vi "加标模块单控对话框.vi"(10 "数组":refnum<vi>[](array[refnum]), 11 "标题":string="加标模块") -> ()   [LabVIEW 2016, in "质控单元.lvlib"]
panel:
  in  "慢速到液位":bool
  in  "排液":bool
  in  "退出":bool
  in  "柱塞泵":bool
  in  "排液":bool
  in  "搅拌":bool
  in  "进样调速":bool
  in  "进样":bool
  in  "停止":bool
  in  "加标启动":bool
  # "手动控制"
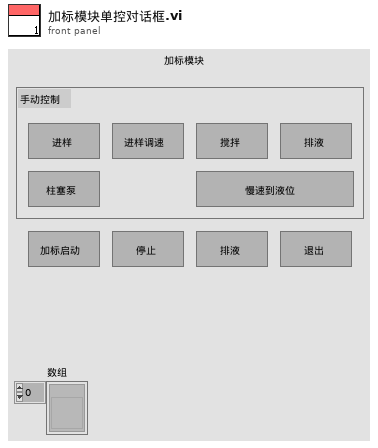
[diagram p1: front panel]
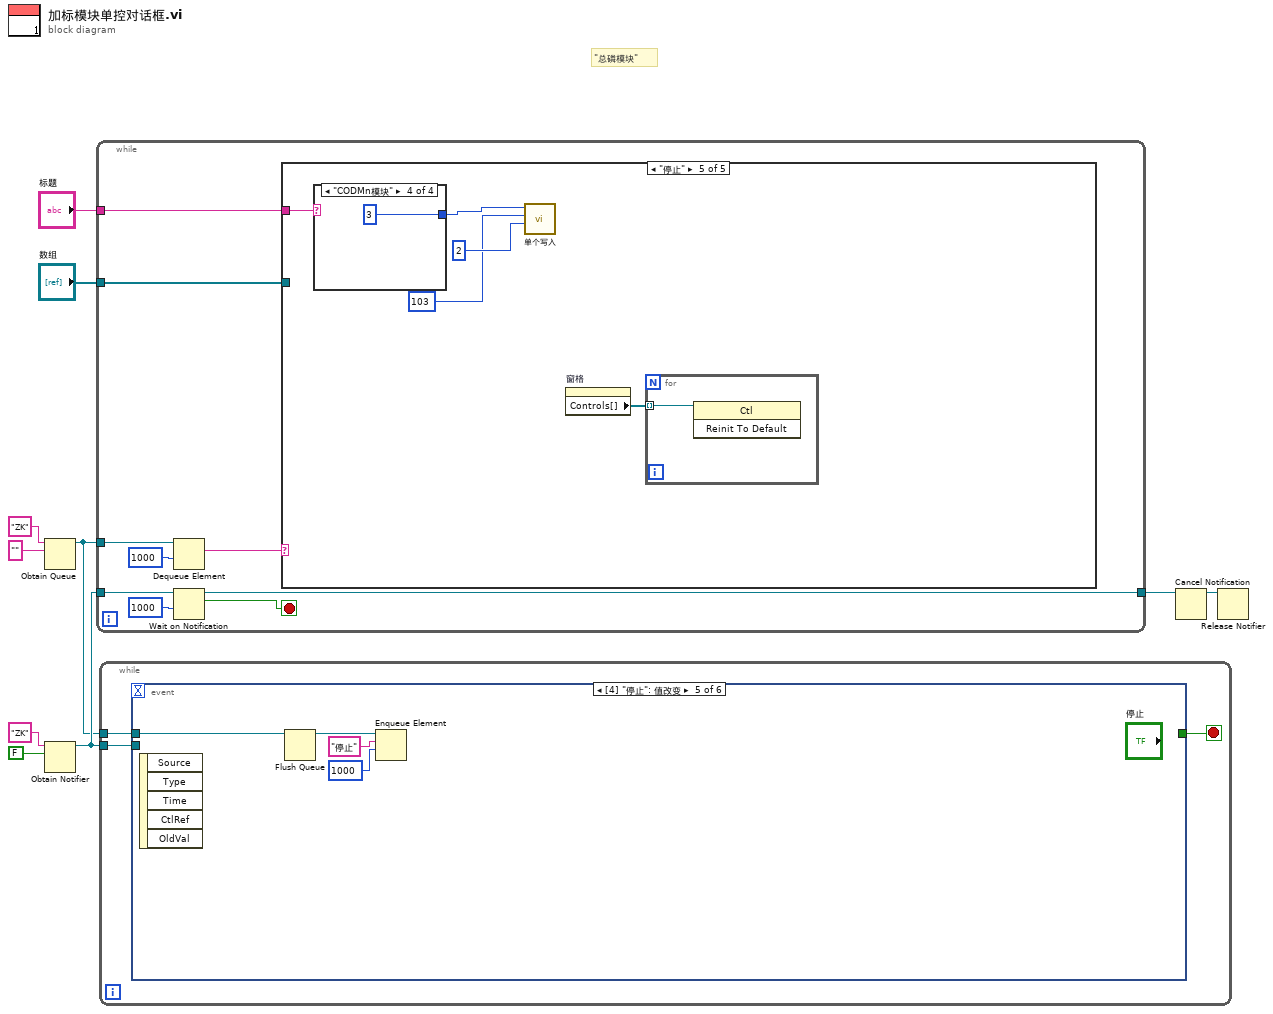
[diagram p0: block diagram]
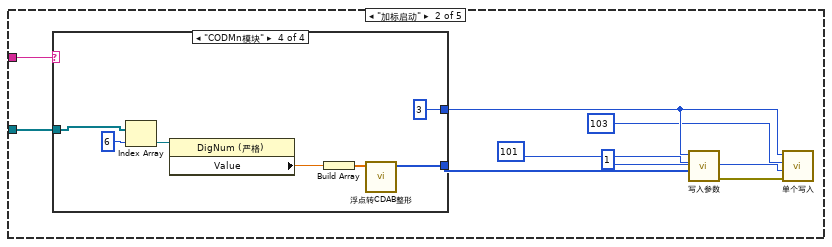
[diagram p3: hidden frame]
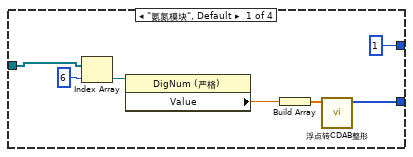
[diagram p4: hidden frame]
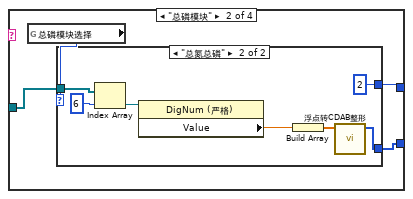
[diagram p5: hidden frame]
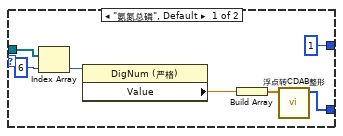
[diagram p6: hidden frame]
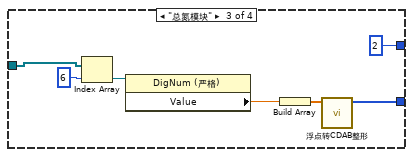
[diagram p7: hidden frame]
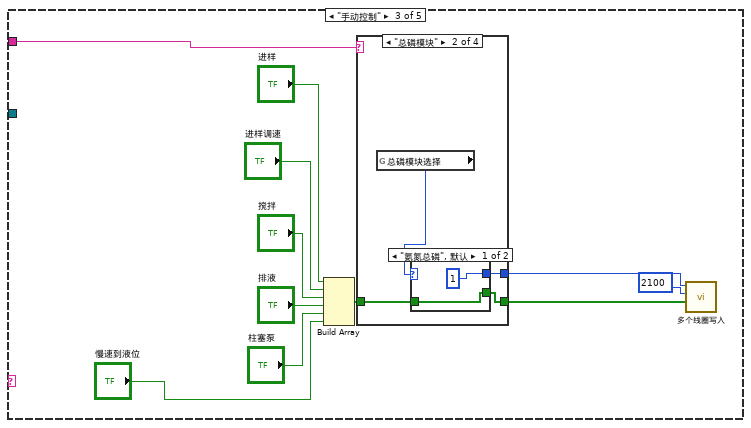
[diagram p8: hidden frame]
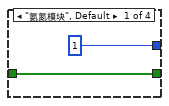
[diagram p9: hidden frame]
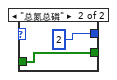
[diagram p10: hidden frame]
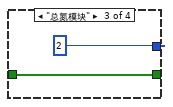
[diagram p11: hidden frame]
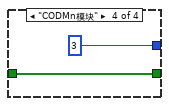
[diagram p12: hidden frame]
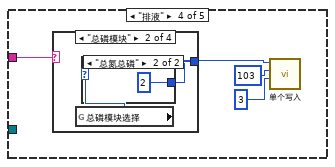
[diagram p13: hidden frame]
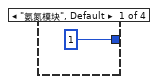
[diagram p14: hidden frame]
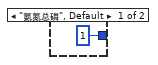
[diagram p15: hidden frame]
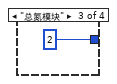
[diagram p16: hidden frame]
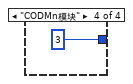
[diagram p17: hidden frame]
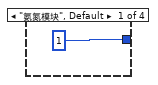
[diagram p18: hidden frame]
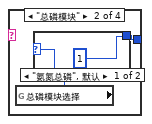
[diagram p19: hidden frame]
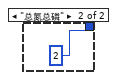
[diagram p20: hidden frame]
diagram:
  # "\"总磷模块\""
  n1 = Obtain Queue(name (unnamed)="ZK" ("名称（未命名）"), element data type="" ("名称（未命名）")) -> (queue out=w3:refnum<queue>)  [unwired: 3 in, 2 out]
  n2 = Obtain Notifier(name (unnamed)="ZK" ("名称（未命名）"), notification data type=FALSE) -> (notifier out=w8:refnum<notifier>)  [unwired: 2 in, 2 out]
  n3 = while {
    tunnel: w8 -> [w19]
    tunnel: [w17] -> w7
    tunnel: w3 -> [w16]
    tunnel: "数组" -> [w11]
    tunnel: "标题" -> [w12]
    stop <- w18 stop-if-true
    n4 = Dequeue Element(queue=w16, timeout in ms (-1)=1000 ("超时毫秒(-1)")) -> (element=w15:string)  [unwired: 1 in, 3 out]
    n5 = Wait on Notification(notifier=w19, timeout in ms (-1)=1000 ("超时毫秒(-1)")) -> (notifier out=w17:refnum<notifier>, notification=w18:bool)  [unwired: 2 in, 2 out]
    n6 = case shown="\"停止\"" w15 {
      tunnel: w12 -> [_ w21 w67 w92 w104]
      tunnel: w11 -> [_ w20 _ _ _]
      frame Default {
      }
      frame "加标启动" {
        n7 = case shown="\"CODMn模块\"" w21 {
          tunnel: w20 -> [w30 w37 w55 w62]
          tunnel: [w29 w36 w54 w61] -> w23
          tunnel: [u8 1 ("Slave ID") w35 u8 2 ("Slave ID") u8 3 ("Slave ID")] -> w27
          frame "氨氮模块", Default {
            n8 = Index Array(array=w30, index=6 ("索引")) -> (element=w34:refnum<vi>)
            n9 = property class="DigNum (严格)"(reference=w34) -> ("Value"=w33:dbl)  [unwired: 1 in, 2 out]
            n10 = Build Array(w33) -> (w32:dbl[])
            n11 = call "浮点转CDAB整形.vi"("浮点数"=w32) -> ("CDAB整形输出"=w29:u16[])  [unwired: 10 in]
          }
          frame "总磷模块" {
            n12 = global read "质控测完标志全局 1.vi" "总磷模块选择"() -> (w38:enum32{"氨氮总磷", "总氮总磷"})
            n13 = case shown="\"总氮总磷\"" w38 {
              tunnel: w37 -> [w39 w48]
              tunnel: [w40 w47] -> w36
              tunnel: [u8 1 ("Slave ID") u8 2 ("Slave ID")] -> w35
              frame "氨氮总磷", Default {
                n14 = Index Array(array=w39, index=6 ("索引")) -> (element=w44:refnum<vi>)
                n15 = property class="DigNum (严格)"(reference=w44) -> ("Value"=w43:dbl)  [unwired: 1 in, 2 out]
                n16 = Build Array(w43) -> (w42:dbl[])
                n17 = call "浮点转CDAB整形.vi"("浮点数"=w42) -> ("CDAB整形输出"=w40:u16[])  [unwired: 10 in]
              }
              frame "总氮总磷" {
                n18 = Index Array(array=w48, index=6 ("索引")) -> (element=w52:refnum<vi>)
                n19 = property class="DigNum (严格)"(reference=w52) -> ("Value"=w51:dbl)  [unwired: 1 in, 2 out]
                n20 = Build Array(w51) -> (w50:dbl[])
                n21 = call "浮点转CDAB整形.vi"("浮点数"=w50) -> ("CDAB整形输出"=w47:u16[])  [unwired: 10 in]
              }
            }
          }
          frame "总氮模块" {
            n22 = Index Array(array=w55, index=6 ("索引")) -> (element=w59:refnum<vi>)
            n23 = property class="DigNum (严格)"(reference=w59) -> ("Value"=w58:dbl)  [unwired: 1 in, 2 out]
            n24 = Build Array(w58) -> (w57:dbl[])
            n25 = call "浮点转CDAB整形.vi"("浮点数"=w57) -> ("CDAB整形输出"=w54:u16[])  [unwired: 10 in]
          }
          frame "CODMn模块" {
            n26 = Index Array(array=w62, index=6 ("索引")) -> (element=w66:refnum<vi>)
            n27 = property class="DigNum (严格)"(reference=w66) -> ("Value"=w65:dbl)  [unwired: 1 in, 2 out]
            n28 = Build Array(w65) -> (w64:dbl[])
            n29 = call "浮点转CDAB整形.vi"("浮点数"=w64) -> ("CDAB整形输出"=w61:u16[])  [unwired: 10 in]
          }
        }
        n30 = call "写入参数.vi"("values"=w23, "starting address"=u16 101, "Slave ID"=w27) -> ("error out"=w22:errorcluster)  [unwired: 8 in]
        n31 = call "单个写入.vi"("Error in"=w22, "value"=u16 1, "address"=u16 103, "Slave ID"=w27) -> ()  [unwired: 7 in, 1 out]
      }
      frame "手动控制" {
        n32 = Build Array("进样", "进样调速", "搅拌", "排液", "柱塞泵", "慢速到液位") -> (w73:bool[])
        n33 = case shown="\"总磷模块\"" w67 {
          tunnel: w73 -> [w79 w82 w88 w91]
          tunnel: [w79 w81 w88 w91] -> w74
          tunnel: [u8 1 ("Slave ID") w80 u8 2 ("Slave ID") u8 3 ("Slave ID")] -> w76
          frame "氨氮模块", Default {
          }
          frame "总磷模块" {
            n34 = global read "质控测完标志全局 1.vi" "总磷模块选择"() -> (w83:enum32{"氨氮总磷", "总氮总磷"})
            n35 = case shown="\"氨氮总磷\", 默认" w83 {
              tunnel: w82 -> [w85 w87]
              tunnel: [w85 w87] -> w81
              tunnel: [u8 1 ("Slave ID") u8 2 ("Slave ID")] -> w80
              frame "氨氮总磷", Default {
              }
              frame "总氮总磷" {
              }
            }
          }
          frame "总氮模块" {
          }
          frame "CODMn模块" {
          }
        }
        n36 = call "多个线圈写入.vi"("values"=w74, "starting address"=u16 2100, "Slave ID"=w76) -> ()  [unwired: 8 in, 1 out]
      }
      frame "排液" {
        n37 = case shown="\"总磷模块\"" w92 {
          tunnel: [u8 1 ("Slave ID") w97 u8 2 ("Slave ID") u8 3 ("Slave ID")] -> w93
          frame "氨氮模块", Default {
          }
          frame "总磷模块" {
            n38 = global read "质控测完标志全局 1.vi" "总磷模块选择"() -> (w98:enum32{"氨氮总磷", "总氮总磷"})
            n39 = case shown="\"总氮总磷\"" w98 {
              tunnel: [u8 1 ("Slave ID") u8 2 ("Slave ID")] -> w97
              frame "氨氮总磷", Default {
              }
              frame "总氮总磷" {
              }
            }
          }
          frame "总氮模块" {
          }
          frame "CODMn模块" {
          }
        }
        n40 = call "单个写入.vi"("value"=u16 3, "address"=u16 103, "Slave ID"=w93) -> ()  [unwired: 8 in, 1 out]
      }
      frame "停止" {
        n41 = case shown="\"CODMn模块\"" w104 {
          tunnel: [u8 1 ("Slave ID") w110 u8 2 ("Slave ID") u8 3 ("Slave ID")] -> w105
          frame "氨氮模块", Default {
          }
          frame "总磷模块" {
            n42 = global read "质控测完标志全局 1.vi" "总磷模块选择"() -> (w111:enum32{"氨氮总磷", "总氮总磷"})
            n43 = case shown="\"氨氮总磷\", 默认" w111 {
              tunnel: [u8 1 ("Slave ID") u8 2 ("Slave ID")] -> w110
              frame "氨氮总磷", Default {
              }
              frame "总氮总磷" {
              }
            }
          }
          frame "总氮模块" {
          }
          frame "CODMn模块" {
          }
        }
        n44 = call "单个写入.vi"("value"=u16 2, "address"=u16 103, "Slave ID"=w105) -> ()  [unwired: 8 in, 1 out]
        n45 = property on="窗格" class="Pane"() -> ("Controls[]"=w103:refnum<vi>[])  [unwired: 2 in, 2 out]
        n46 = for {
          tunnel: w103 -> [w108] mode=indexing
          n47 = invoke class="Ctl" method="Reinit To Default"(reference=w108) -> ()  [unwired: 2 in, 3 out]
        }
      }
    }
  }
  n48 = while {
    tunnel: w8 -> [w117]
    tunnel: w3 -> [w116]
    stop <- w118 stop-if-true
    n49 = event shown="[4] \"停止\": 值改变" {
      selector: _ -> [_ _ _ _ _ _]
      dyn-events: _ -> [_ _ _ _ _ _]
      timeout: _ -> [_ _ _ _ _ _]
      tunnel: [_ _ _ _ _ TRUE] -> w118
      tunnel: w117 -> [_ _ _ _ _ w134]
      tunnel: w116 -> [_ w121 w122 w125 w130 w133]
      event Timeout {
        n50 = event-data() -> ()  [unwired: 1 in, 3 out]
      }
      event "加标启动": Value Change {
        n51 = event-data() -> ()  [unwired: 1 in, 4 out]
        n52 = Enqueue Element(queue=w121, element="加标启动" ("元素"), timeout in ms (-1)=1000 ("超时毫秒(-1)")) -> ()  [unwired: 1 in, 3 out]
      }
      event "进样", "进样调速", "搅拌", "排液", "柱塞泵", "慢速到液位": Value Change {
        n53 = event-data() -> ()  [unwired: 1 in, 5 out]
        n54 = Enqueue Element(queue=w122, element="手动控制" ("元素"), timeout in ms (-1)=1000 ("超时毫秒(-1)")) -> ()  [unwired: 1 in, 3 out]
      }
      event "排液": Value Change {
        n55 = event-data() -> ()  [unwired: 1 in, 6 out]
        n56 = Enqueue Element(queue=w125, element="排液" ("元素"), timeout in ms (-1)=1000 ("超时毫秒(-1)")) -> ()  [unwired: 1 in, 3 out]
      }
      event "停止": Value Change {
        n57 = event-data() -> ()  [unwired: 1 in, 5 out]
        n58 = Flush Queue(queue=w130) -> (queue out=w129:refnum<queue>)  [unwired: 1 in, 2 out]
        n59 = Enqueue Element(queue=w129, element="停止" ("元素"), timeout in ms (-1)=1000 ("超时毫秒(-1)")) -> ()  [unwired: 1 in, 3 out]
      }
      event "退出": Value Change; Panel Close {
        n60 = event-data() -> ()  [unwired: 1 in, 3 out]
        n61 = Send Notification(notification=TRUE ("通知"), notifier=w134) -> ()  [unwired: 1 in, 2 out]
        n62 = Flush Queue(queue=w133) -> (queue out=w132:refnum<queue>)  [unwired: 1 in, 2 out]
        n63 = Two Button Dialog(message="请确认是否退出，退出仪器将停止运行" ("消息"), 1:"N" ("F按钮名称（“取消”）"), 2:"Y" ("T按钮名称（“确定”）")) -> (T button?=w136:bool)
        n64 = case shown="真" w136 {
          tunnel: w132 -> [_ w141]
          frame False {
          }
          frame True {
            n65 = property on="窗格" class="Pane"() -> ("Controls[]"=w144:refnum<vi>[])  [unwired: 2 in, 2 out]
            n66 = Enqueue Element(queue=w141, element="停止" ("元素"), timeout in ms (-1)=1000 ("超时毫秒(-1)")) -> ()  [unwired: 1 in, 3 out]
            n67 = for {
              tunnel: w144 -> [w145] mode=indexing
              n68 = invoke class="Ctl" method="Reinit To Default"(reference=w145) -> ()  [unwired: 2 in, 3 out]
            }
          }
        }
      }
    }
  }
  n69 = Cancel Notification(0:w7) -> (8:w6:refnum<notifier>)  [unwired: 1 in, 2 out]
  n70 = Release Notifier(notifier=w6) -> ()  [unwired: 2 in, 3 out]
